vi "libssh2_sftp_seek64.vi"(8 "error in (no error)":errorcluster, 10 "offset":u64, 11 "sftp handle":T1) -> (0 "error out":errorcluster)   [LabVIEW 2013, in "libssh2.lvlib"]
doc: "Set the file position of a file handle."
uses:
  libssh2.lvlib
  SFTP Handle Refnum.ctl
  Not An SFTP Handle Refnum.vi
  <vilib>/Utility/error.llb/Error Cluster From Error Code.vi
  Global Settings.vi
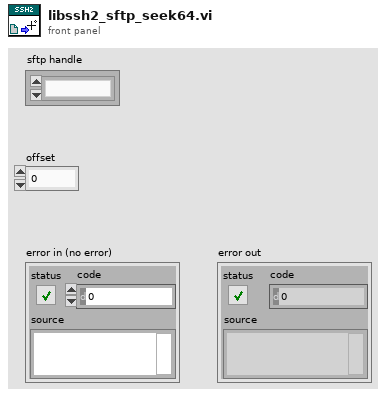
[diagram p1: front panel]
types:
  T1 = typedef "libssh2.lvlib/SFTP Handle Refnum.ctl" = refnum<k1>
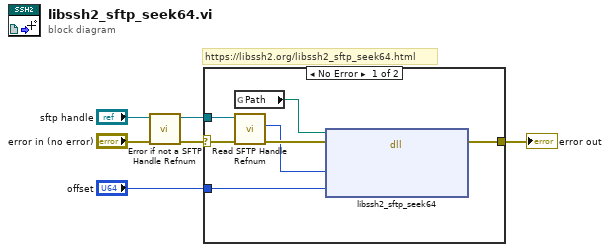
[diagram p0: block diagram]
diagram:
  # "https://libssh2.org/libssh2_sftp_seek64.html"
  n1 = call "Error if not a SFTP Handle Refnum.vi"("error in (no error)"="error in (no error)", "sftp handle"="sftp handle") -> ("error out"=w5:errorcluster, "sftp handle out"=w4:T1)  [unwired: 8 in]
  n2 = case shown="No Error" w5 {
    selector: w5 -> [w12 w14]
    tunnel: w4 -> [w11 _]
    tunnel: [w8 w14] -> w3
    tunnel: "offset" -> [w7 _]
    frame No Error {
      n3 = global read "Global Settings.vi" "Path"() -> (w13:path)
      n4 = call "Read SFTP Handle Refnum.vi"("error in (no error)"=w12, "sftp handle"=w11) -> ("error out"=w10:errorcluster, "LIBSSH2_SFTP_HANDLE*"=w9:u64)  [unwired: 8 in]
      n5 = dll-call lib="?" fn="libssh2_sftp_seek64"(path in=w13, error in=w10, "handle"=w9, "offset"=w7) -> (error out=w8:errorcluster)  [unwired: 4 in, 1 out]
    }
    frame Error {
    }
  }
  "error out" <- w3
